vi "Device ID to Name.vi"(8 "Error In":errorcluster, 9 "Device Index":i32, 10 "Family Index":i32, 11 "LINX Device Config":T1) -> (0 "Error Out":errorcluster, 2 "Device Name":string, 3 "LINX Device Config":T1)   [LabVIEW 2011, in "LMH-LINX.lvlib"]
doc: "Get the device name from the device family and device ID."
uses:
  LMH-LINX.lvlib
  Device/Type Defs/LINX Device Config.ctl
  Type Defs/Interface.ctl
  Device/Type Defs/TCP Config.ctl
  Device/Type Defs/Channels.ctl
  Type Defs/All Firmware Data FGV States.ctl
  Device/Device.lvlib
panel:
  out "Family Index":i32
  out "Device Index":i32
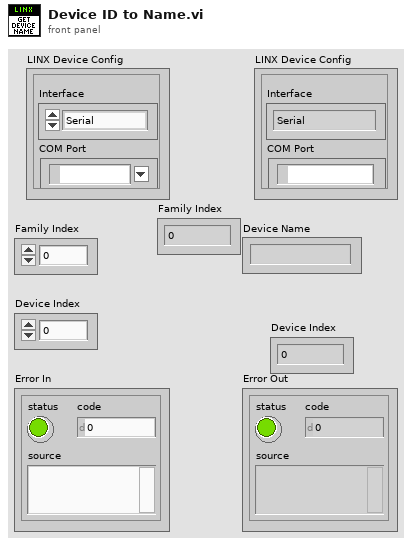
[diagram p1: front panel]
types:
  T1 = typedef "LMH-LINX.lvlib/Device.lvlib/LINX Device Config.ctl" = cluster{"Interface":T2, "COM Port":refnum<visa-resource-name>, "TCP Configuration":T3, "Device Family":u8, "Device ID":u8, "Device Name":string, "TCP Ref":refnum<k5>, "Channels":T4}
  T2 = typedef "LMH-LINX.lvlib/Interface.ctl" = enum16{"Serial", "TCP"}
  T3 = typedef "LMH-LINX.lvlib/Device.lvlib/TCP Config.ctl" = cluster{"IP Address":string, "Port":u16}
  T4 = typedef "LMH-LINX.lvlib/Channels.ctl" = cluster{"DI":u8[], "DO":u8[], "AI":u8[], "AO":u8[], "PWM":u8[], "QE":u8[], "UART":u8[], "I2C 2":u8[], "SPI":u8[], "CAN":u8[], "Servo":u8[], "AI Ref (V)":dbl, "AI Resolution (Bits)":u8, "AO Ref (V)":dbl, "AO Resolution (Bits)":u8}
  T5 = typedef "LMH-LINX.lvlib/All Firmware Data FGV States.ctl" = enum16{"Set", "Get"}
  T6 = typedef "LMH-LINX.lvlib/Device Data.ctl" = cluster{"Family ID":i32, "Family Name":string, "Device ID":i32, "Device Name":string, "Firmware Program Interfaces":string[], "Path":path}
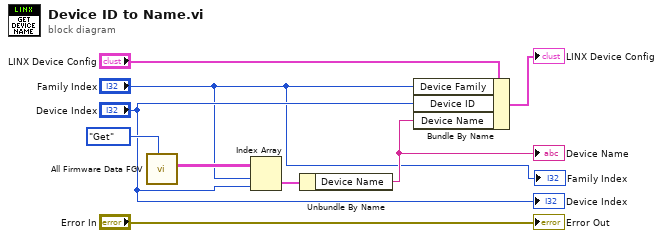
[diagram p0: block diagram]
diagram:
  n1 = call "All Firmware Data FGV.vi"("All Firmware Data FGV States"=All_Firmware_Data_FGV_States."Get") -> ("Devices"=w5:T6[][])  [unwired: 7 in, 3 out]
  n2 = Index Array(array=w5, index (row)="Family Index", index (col)="Device Index") -> (element=w4:T6)
  n3 = Unbundle By Name(w4) -> ("Device Name"=w3:string)
  "Device Name" <- w3
  n4 = Bundle By Name(cluster="LINX Device Config", "Device Family"="Family Index", "Device ID"="Device Index", "Device Name"=w3) -> (→"LINX Device Config":T1)
  "Error Out" <- "Error In"
  "Device Index" <- "Device Index"
  "Family Index" <- "Family Index"
